vi "SwitchPage.vi"(8 "error in (no error)":errorcluster, 10 "Page":string, 11 "ViewMgr in":refnum<class "ViewMgr.lvclass">) -> (0 "error out":errorcluster, 3 "ViewMgr out":refnum<class "ViewMgr.lvclass">)   [LabVIEW 2020, in "CSM-TagDBDisplayContainer.lvlib" / "ViewMgr.lvclass"]
uses:
  ViewMgr.lvclass
  ViewMgr.lvclass/ViewMgr.ctl
  CSM-TagDBDisplayContainer.lvlib
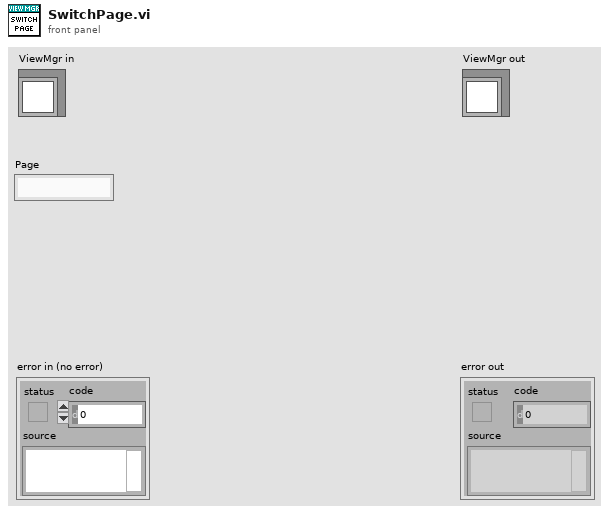
[diagram p1: front panel]
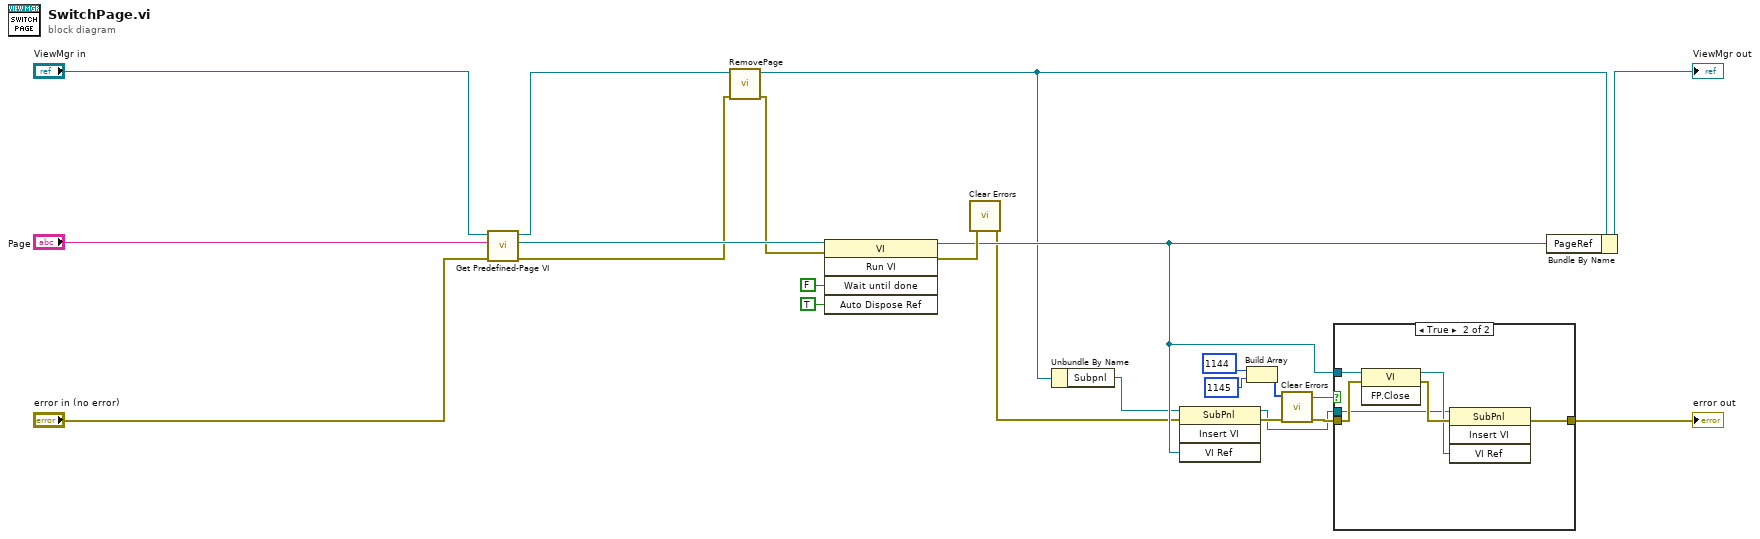
[diagram p0: block diagram]
diagram:
  n1 = call "Get Predefined-Page VI.vi"("error in (no error)"="error in (no error)", "Page"="Page", "ViewMgr in"="ViewMgr in") -> ("error out"=w5:errorcluster, "PageVI Ref"=w22:refnum<vi>, "ViewMgr out"=w8:refnum<class "ViewMgr.lvclass">)  [unwired: 6 in]
  n2 = call "RemovePage.vi"("error in (no error)"=w5, "ViewMgr in"=w8) -> ("error out"=w6:errorcluster, "ViewMgr out"=w2:refnum<class "ViewMgr.lvclass">)  [unwired: 8 in]
  n3 = invoke class="VI" method="Run VI"(reference=w22, error in=w6, "Wait until done"=FALSE ("Wait Until Done"), "Auto Dispose Ref"=TRUE ("Auto Dispose Reference")) -> (reference out=w14:refnum<vi>, error out=w18:errorcluster)  [unwired: 1 in, 3 out]
  n4 = call <vilib>:"Clear Errors.vi"("error in (no error)"=w18) -> ("error out"=w7:errorcluster)  [unwired: 5 in, 1 out]
  n5 = Unbundle By Name(w2) -> ("Subpnl"=w1:refnum<vi>)
  n6 = invoke class="SubPnl" method="Insert VI"(reference=w1, error in=w7, "VI Ref"=w14) -> (reference out=w12:refnum<vi>, error out=w17:errorcluster)  [unwired: 1 in, 2 out]
  n7 = Build Array(1144 ("specific error code to clear (0: all)"), 1145 ("specific error code to clear (0: all)")) -> (w11:i32[])
  n8 = call <vilib>:"Clear Errors.vi"("error in (no error)"=w17, "specific error code to clear (0: all)"=w11) -> ("error out"=w13:errorcluster, "specific error cleared?"=w15:bool)  [unwired: 8 in]
  n9 = case shown="True" w15 {
    tunnel: w14 -> [_ w30]
    tunnel: w13 -> [w24 w28]
    tunnel: [w24 w27] -> w3
    tunnel: w12 -> [_ w25]
    frame False {
    }
    frame True {
      n10 = invoke class="VI" method="FP.Close"(reference=w30, error in=w28) -> (reference out=w26:refnum<vi>, error out=w29:errorcluster)  [unwired: 1 in, 1 out]
      n11 = invoke class="SubPnl" method="Insert VI"(reference=w25, error in=w29, "VI Ref"=w26) -> (error out=w27:errorcluster)  [unwired: 1 in, 3 out]
    }
  }
  "error out" <- w3
  n12 = Bundle By Name(cluster=w2, "PageRef"=w14) -> (→"ViewMgr out":refnum<class "ViewMgr.lvclass">)
